vi "StartCPUMonitoring.vi"(8 "error in (no error)":errorcluster, 9 "CPU Monitoring On (T)":bool=TRUE, 10 "port number (3363)":u32, 11 "machine name (\"\":  open local reference)":string) -> (0 "error out":errorcluster)   [LabVIEW 2010, in "kevLib2010.lvlib"]
uses:
  kevLib2010.lvlib
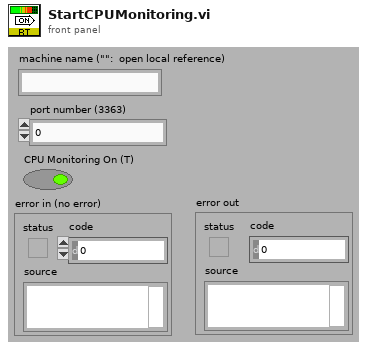
[diagram p1: front panel]
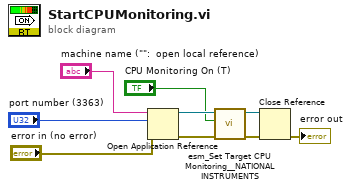
[diagram p0: block diagram]
diagram:
  n1 = Open Application Reference(8:"error in (no error)", 10:"port number (3363)", 11:"machine name (\"\":  open local reference)") -> (0:w9:errorcluster, 3:w8:refnum<vi>)  [unwired: 1 in]
  n2 = call "esm_Set Target CPU Monitoring__NATIONAL INSTRUMENTS.vi"("error in (no error)"=w9, "CPU Monitoring On"="CPU Monitoring On (T)", "application reference"=w8) -> ("error out"=w6:errorcluster, "application reference out"=w7:refnum<vi>)  [unwired: 7 in]
  n3 = Close Reference(reference=w7, error in (no error)=w6) -> (error out=→"error out":errorcluster)
